vi "Destroy.vi"(0 "reference in":refnum<class "Map.lvclass">, 5 "error in (no error)":errorcluster) -> (14 "reference out":refnum<class "Map.lvclass">, 19 "error out":errorcluster)   [LabVIEW 2020, in "Map.lvclass"]
doc: "This VI destroys the Map Object"
uses:
  Map.lvclass
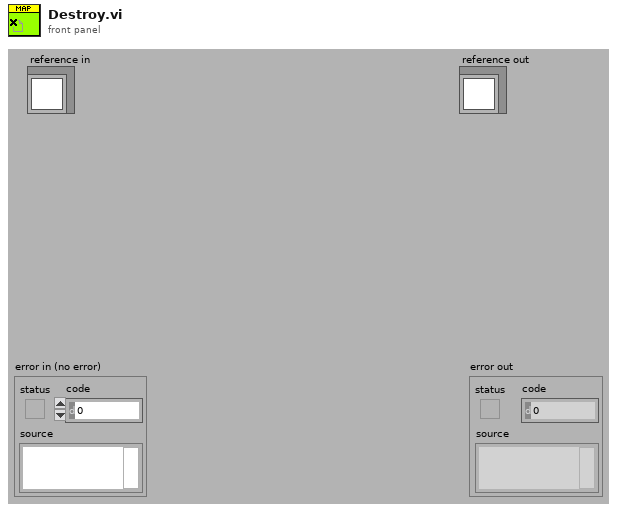
[diagram p1: front panel]
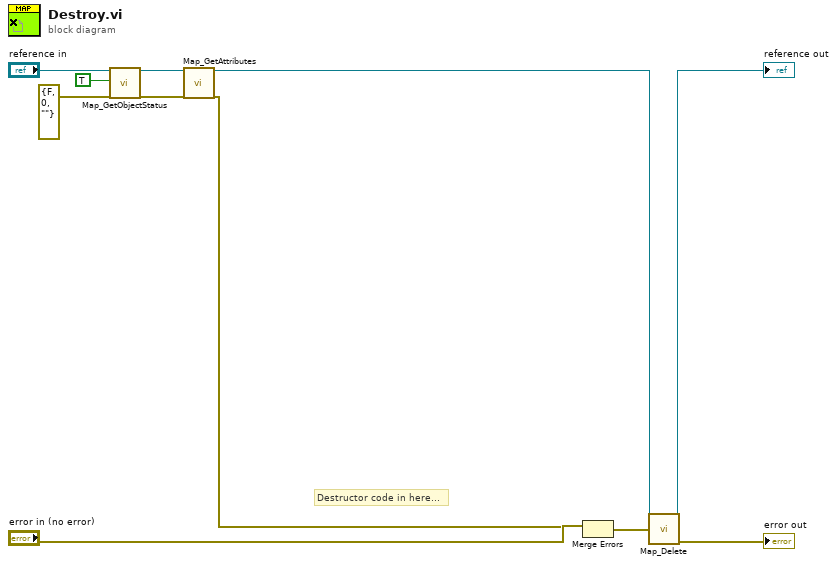
[diagram p0: block diagram]
diagram:
  # "Destructor code in here..."
  n1 = call "Map_GetObjectStatus.vi"("reference in"="reference in", "Simple Info"=TRUE, "error in (no error)"=errorcluster {"status"=FALSE, "code"=0, "source"=""}) -> ("reference out"=w5:refnum<class "Map.lvclass">, "error out"=w2:errorcluster)  [unwired: 15 out]
  n2 = call "Map_GetAttributes.vi"("reference in"=w5, "error in (no error)"=w2) -> ("reference out"=w9:refnum<class "Map.lvclass">, "error out"=w7:errorcluster)  [unwired: 16 out]
  n3 = Merge Errors("error in (no error)", w7) -> (w8:errorcluster)
  n4 = call "Map_Delete.vi"("reference in"=w9, "error in (no error)"=w8) -> ("reference out"=→"reference out":refnum<class "Map.lvclass">, "error out"=→"error out":errorcluster)  [unwired: 1 in, 15 out]
